vi "EnabledChannelArray.vi"(10 "Channel1":i16, 11 "Channel0":i16) -> (3 "EnabledChannels":string[](array[string]))   [LabVIEW 2020, in "PicoscopeV2.lvclass"]
uses:
  PicoscopeV2.lvclass
  shared/OnOffTypeDef.ctl
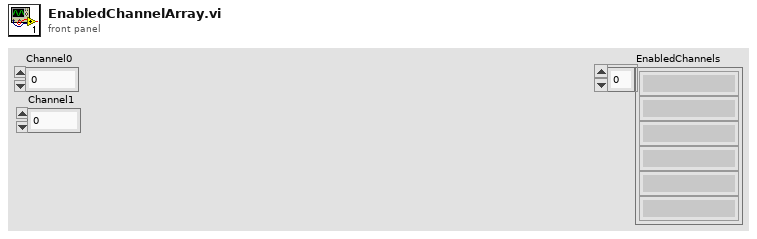
[diagram p1: front panel]
types:
  T1 = typedef "OnOffTypeDef.ctl" = enum16{"off", "on"}
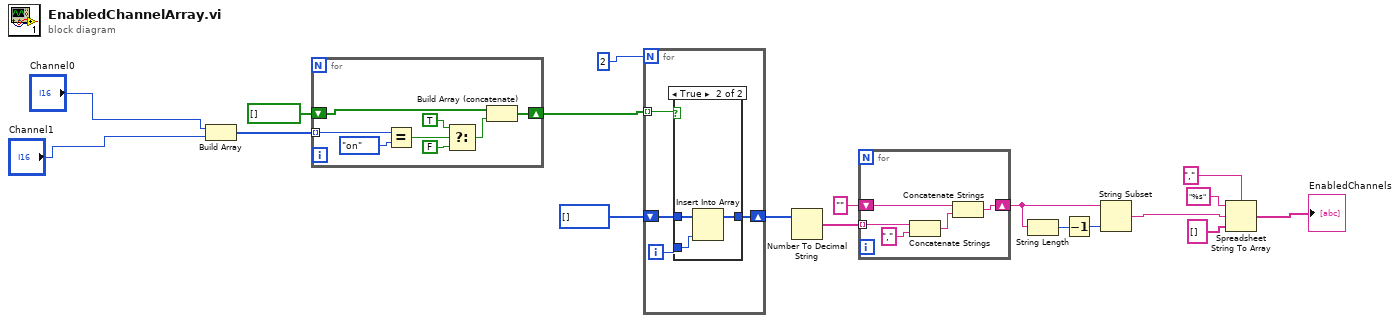
[diagram p0: block diagram]
diagram:
  n1 = Build Array("Channel0", "Channel1") -> (w8:i16[])
  n2 = for {
    tunnel: w8 -> [w26] mode=indexing
    shift-right: [w19] -> w6
    shift-left: bool[] [] -> [w21]
    n3 = Equal?(x=w26, y=OnOffTypeDef."on" ("Settings.channelenabled.Channel0")) -> (x = y?=w24:bool)
    n4 = Select(t=TRUE, s=w24, f=FALSE) -> (s? t:f=w20:bool)
    n5 = Build Array (concatenate)(w21, w20) -> (w19:bool[])
  }
  n6 = for {
    N: 2 -> [_]
    tunnel: w6 -> [w30] mode=indexing
    shift-right: [w28] -> w4
    shift-left: i32[] [] -> [w29]
    i -> [w27]
    n7 = case shown="True" w30 {
      tunnel: [w31 w34] -> w28
      tunnel: w29 -> [w31 w33]
      tunnel: w27 -> [_ w32]
      frame False {
      }
      frame True {
        n8 = Insert Into Array(array=w33, new element=w32) -> (w34:i32[])  [unwired: 1 in]
      }
    }
  }
  n9 = Number To Decimal String(number=w4) -> (decimal integer string=w17:string[])  [unwired: 1 in]
  n10 = for {
    tunnel: w17 -> [w38] mode=indexing
    shift-right: [w37] -> w16
    shift-left: "" -> [w36]
    n11 = Concatenate Strings(w38, "," ("string")) -> (w35:string)
    n12 = Concatenate Strings(w36, w35) -> (w37:string)
  }
  n13 = String Length(string=w16) -> (length=w14:i32)
  n14 = Decrement(x=w14) -> (x-1=w15:i32)
  n15 = String Subset(string=w16, length (rest)=w15) -> (substring=w18:string)  [unwired: 1 in]
  n16 = Spreadsheet String To Array(delimiter (Tab)=",", format string="%s", spreadsheet string=w18, array type (2D Dbl)=string[] []) -> (array=→"EnabledChannels":string[])
